vi "find possible directions.vi"(9 "Drone":T3, 11 "Field":T2[][](array[typedef])) -> (1 "possible directions":T1[](array[typedef]) items=["^", "^>", ">", "V>", "V", "<V", "<", "<^"], 3 "move matrix":bool[][](array[boolean]))   [LabVIEW 2009]
uses:
  Drone data.ctl
  square.ctl
  direction.ctl
panel:
  in  "radius":i32=1
  # "Currently only works with a radius of 1 (due to unwrapping algorithm)"
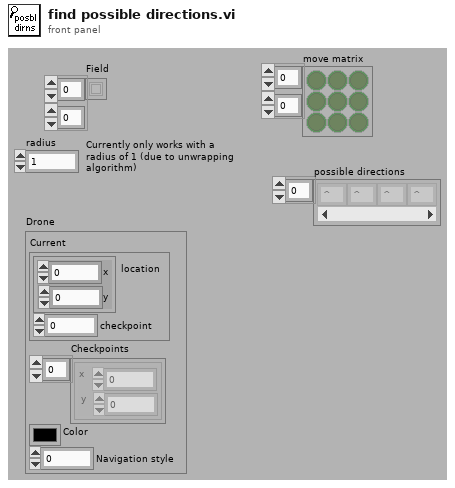
[diagram p1: front panel]
types:
  T1 = typedef "direction.ctl" = i8
  T2 = typedef "square.ctl" = u8
  T3 = typedef "Drone data.ctl" = cluster{"Current":cluster{"location":cluster{"x":i16, "y":i16}, "checkpoint":i32}, "Checkpoints":cluster{"x":i16, "y":i16}[], "Color":u32, "Navigation style":i32}
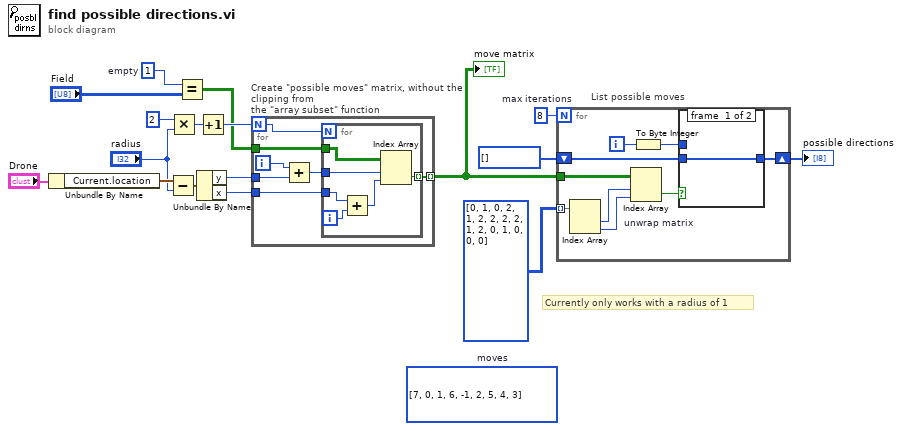
[diagram p0: block diagram]
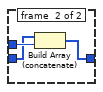
[diagram p2: hidden frame]
diagram:
  w1 = T2 1  # empty
  w11 = 8  # max iterations
  w13 = T1[] [] items=["O"=-1, "^"=0, "^>"=1, ">"=2, "V>"=3, "V"=4, "<V"=5, "<"=6, "<^"=7]
  (unwired) T1[][] [[7, 0, 1], [6, -1, 2], [5, 4, 3]] items=["O"=-1, "^"=0, "^>"=1, ">"=2, "V>"=3, "V"=4, "<V"=5, "<"=6, "<^"=7]  # moves
  # "Currently only works with a radius of 1"
  n1 = Unbundle By Name("Drone") -> ("Current.location"=w16:cluster{"x":i16, "y":i16})
  n2 = Subtract(x=w16, y="radius") -> (x-y=w7:cluster{"x":i32, "y":i32})
  n3 = Multiply(x=2, y="radius") -> (x*y=w8:i32)
  n4 = Equal?(x=w1, y="Field") -> (x = y?=w3:bool[][])
  n5 = Unbundle By Name(w7) -> ("y"=w4:i32, "x"=w5:i32)
  n6 = Increment(x=w8) -> (x+1=w6:i32)
  n7 = for "Create \"possible moves\" matrix, without the clipping from\nthe \"array subset\" function" {
    N: w6 -> [w24]
    tunnel: w3 -> [w23]
    tunnel: w5 -> [w22]
    tunnel: w4 -> [w21]
    tunnel: [w18] -> w14 mode=indexing
    i -> [w20]
    n8 = Add(x=w20, y=w21) -> (x+y=w19:i32)
    n9 = for {
      N: w24 -> [_]
      tunnel: w23 -> [w28]
      tunnel: w22 -> [w29]
      tunnel: w19 -> [w27]
      tunnel: [w25] -> w18 mode=indexing
      i -> [w30]
      n10 = Add(x=w29, y=w30) -> (x+y=w26:i32)
      n11 = Index Array(array=w28, index (row)=w27, index (col)=w26) -> (element=w25:bool)
    }
  }
  "move matrix" <- w14
  n12 = for "List possible moves" {
    N: w11 -> [_]
    tunnel: i32[][] [[0, 1], [0, 2], [1, 2], [2, 2], [2, 1], [2, 0], [1, 0], [0, 0]] -> [w39] mode=indexing
    tunnel: w14 -> [w38]
    shift-right: [w32] -> w12
    shift-left: w13 -> [w34]
    i -> [w35]
    n13 = Index Array(array=w39) -> (element #1=w37:i32, element #2=w36:i32)  [unwired: 2 in]
    n14 = Index Array "unwrap matrix"(array=w38, index (row)=w37, index (col)=w36) -> (element=w31:bool)
    n15 = To Byte Integer(number=w35) -> (8bit integer=w33:i8)
    n16 = case shown="False" w31 {
      tunnel: w33 -> [_ w43]
      tunnel: w34 -> [w40 w42]
      tunnel: [w40 w41] -> w32
      frame #0 {
      }
      frame #1 {
        n17 = Build Array (concatenate)(w42, w43) -> (w41:T1[])
      }
    }
  }
  "possible directions" <- w12
